vi "READ_SUPPLY.vi"(0 "VISA resource name":refnum<visa-resource-name>, 5 "Board address":u8, 7 "NChannels":u8, 11 "error in (no error)":errorcluster) -> (6 "VMon values (V)":dbl[](array[numeric]) format="%.1f", 8 "IMon values (uA)":dbl[](array[numeric]) format="%.2f", 15 "error out":errorcluster)   [LabVIEW 2012]
uses:
  <instrlib>/CAEN PSM/CAEN PSM.lvlib
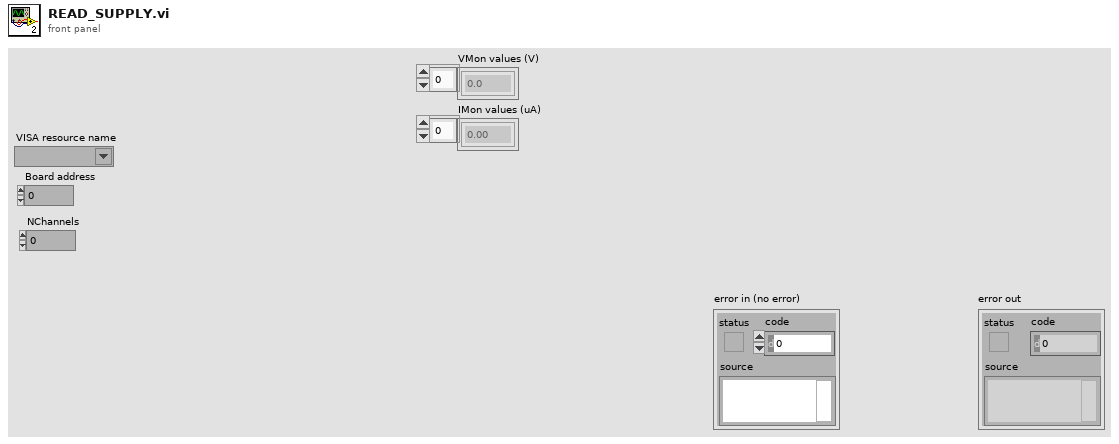
[diagram p1: front panel]
types:
  T1 = cluster{"VISA resource name":refnum<visa-resource-name>, "Board address":u8, "NChannels":u8}
  T2 = typedef "CAEN PSM.lvlib/BoardHandle.ctl" = cluster{"VISA resource name":refnum<visa-resource-name>, "Board address":u8, "NChannels":u8}
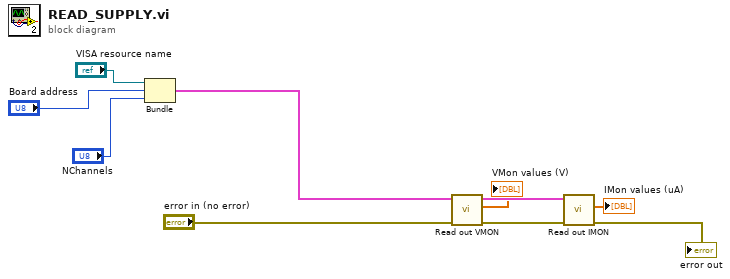
[diagram p0: block diagram]
diagram:
  n1 = Bundle("VISA resource name"="VISA resource name", "Board address"="Board address", "NChannels"="NChannels") -> (w4:T1)  [unwired: 1 in]
  n2 = call <instrlib>:"Read out VMON.vi"("error in (no error)"="error in (no error)", "BoardHandle"=w4) -> ("error out"=w9:errorcluster, "VMon values (V)"=→"VMon values (V)":dbl[], "BoardHandle out"=w10:T2)  [unwired: 7 in]
  n3 = call <instrlib>:"Read out IMON.vi"("error in (no error)"=w9, "BoardHandle"=w10) -> ("error out"=→"error out":errorcluster, "IMon values (uA)"=→"IMon values (uA)":dbl[])  [unwired: 6 in, 2 out]
